vi "Msg.Noti.Send.vi"(8 "Error (in)":errorcluster, 9 "Data":variant, 10 "Message":string, 11 "Msg.Refs":T1) -> (0 "Error (out)":errorcluster, 3 "Msg.Refs (out)":T1)   [LabVIEW 2023]
uses:
  Msg.Data.ctl
  Msg.Event.Ref.ctl
  Msg.Event.RegRef.ctl
  Msg.Q.Ref.ctl
  Msg.Noti.Ref.ctl
  Msg.Refs.ctl
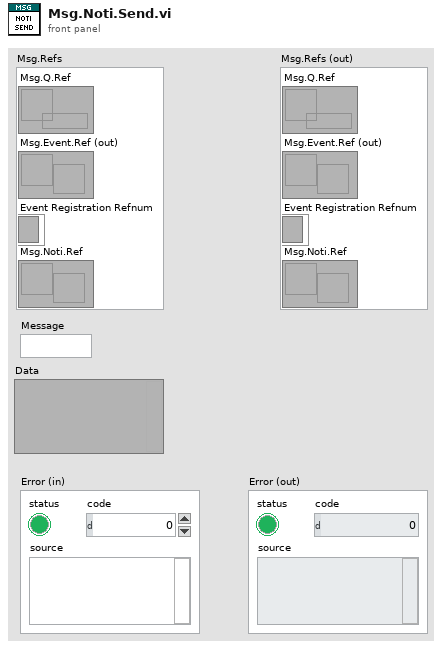
[diagram p1: front panel]
types:
  T1 = typedef "Msg.Refs.ctl" = cluster{"Msg.Q.Ref":T2, "Msg.Event.Ref (out)":T3, "Event Registration Refnum":T4, "Msg.Noti.Ref":T5}
  T2 = typedef "Msg.Q.Ref.ctl" = refnum<queue>
  T3 = typedef "Msg.Event.Ref.ctl" = refnum<user-event>
  T4 = typedef "Msg.Event.RegRef.ctl" = refnum<event-registration>
  T5 = typedef "Msg.Noti.Ref.ctl" = refnum<notifier>
  T6 = typedef "Msg.Data.ctl" = cluster{"Message":string, "Data":variant}
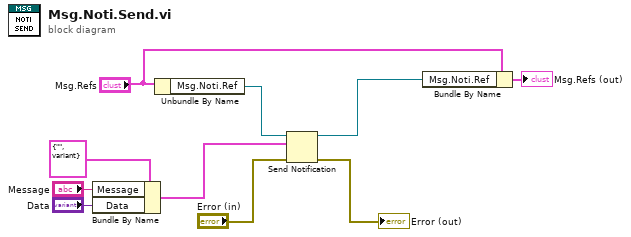
[diagram p0: block diagram]
diagram:
  n1 = Bundle By Name(cluster=T6 {"Message"="", "Data"=variant} ("Msg.Q.Data"), "Message"="Message", "Data"="Data") -> (w8:T6)
  n2 = Unbundle By Name("Msg.Refs") -> ("Msg.Noti.Ref"=w4:T5)
  n3 = Send Notification(notification=w8, notifier=w4, error in (no error)="Error (in)") -> (notifier out=w3:T5, error out=→"Error (out)":errorcluster)
  n4 = Bundle By Name(cluster="Msg.Refs", "Msg.Noti.Ref"=w3) -> (→"Msg.Refs (out)":T1)
